vi "string array manage.vi"(6 "pattern IN":string=".+?\\(.+?\\)", 7 "actions":T1=enum."match pattern", 9 "Array 2 IN":string[](array[string])=["frequency (Hz)", "Cs/T (J/K^2)", "Ts (K)", "Tr (K)", "Cs (J/K)", "Cr (J/K)", "Ks (W/K)", "Kr (W/K)", "Rs-therm (Ohm)", "Rr-therm (Ohm)", "Cr/T (J/K^2)", "dlogR/dlogT -- S  (a.u.)", "tau (s)", "tan(phi) (a.u)", "Ts,ac (K)", "Tr,ac (K)", "Hs,ac,out (V)", "Offset,dc,out (V)", "Stherm,ac,out (V)", "Rtherm,ac,out (V)", "CV1 -- Re (V)", "CV1 -- Im (V)", "DV2 -- Re (V)", "DV2 -- Im (V)", "AV2 -- Re (V)", "AV2 -- Im (V)", "LakeShore 336 (12) A", "LakeShore 336 (12) B", "LakeShore 336 (12) C", "LakeShore 336 (12) D", "field (T)"], 10 "Array 1 IN":string[](array[string])=["Time", "frequency (Hz)", "Cs/T (J/K^2)", "Ts (K)", "Tr (K)", "Cs (J/K)", "Cr (J/K)", "Ks (W/K)", "Kr (W/K)", "Rs-therm (Ohm)", "Rr-therm (Ohm)", "Cr/T (J/K^2)", "dlogR/dlogT -- S  (a.u.)", "tau (s)", "tan(phi) (a.u)", "Ts,ac (K)", "Tr,ac (K)", "Hs,ac,out (V)", "Offset,dc,out (V)", "Stherm,ac,out (V)", "Rtherm,ac,out (V)", "CV1 -- Re (V)", "CV1 -- Im (V)", "DV2 -- Re (V)", "DV2 -- Im (V)", "AV2 -- Re (V)", "AV2 -- Im (V)", "LakeShore 336 (12) A", "LakeShore 336 (12) B", "LakeShore 336 (12) C", "LakeShore 336 (12) D", "pos", "field (T)"]) -> (1 "Array 2 OUT":string[](array[string]), 2 "Array 1 OUT":string[](array[string])=["frequency (Hz)", "Cs/T (J/K^2)", "Ts (K)", "Tr (K)", "Cs (J/K)", "Cr (J/K)", "Ks (W/K)", "Kr (W/K)", "Rs-therm (Ohm)", "Rr-therm (Ohm)", "Cr/T (J/K^2)", "dlogR/dlogT -- S  (a.u.)", "tau (s)", "tan(phi) (a.u)", "Ts,ac (K)", "Tr,ac (K)", "Hs,ac,out (V)", "Offset,dc,out (V)", "Stherm,ac,out (V)", "Rtherm,ac,out (V)", "CV1 -- Re (V)", "CV1 -- Im (V)", "DV2 -- Re (V)", "DV2 -- Im (V)", "AV2 -- Re (V)", "AV2 -- Im (V)", "LakeShore 336 (12) A", "LakeShore 336 (12) B", "LakeShore 336 (12) C", "LakeShore 336 (12) D", "field (T)"])   [LabVIEW 2021]
uses:
  string array manage control.ctl
  6d6d019a-d48c-a744-8711-00c2e699bb64.vi
  <vilib>/regexp/Match Regular Expression.xnode
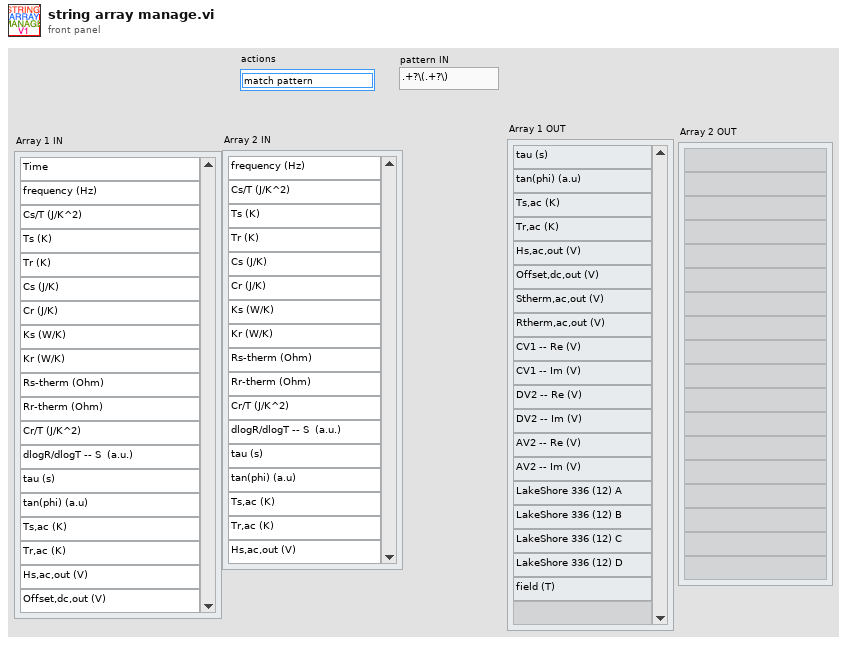
[diagram p1: front panel]
types:
  T1 = typedef "string array manage control.ctl" = enum16{"intersection", "match pattern"}
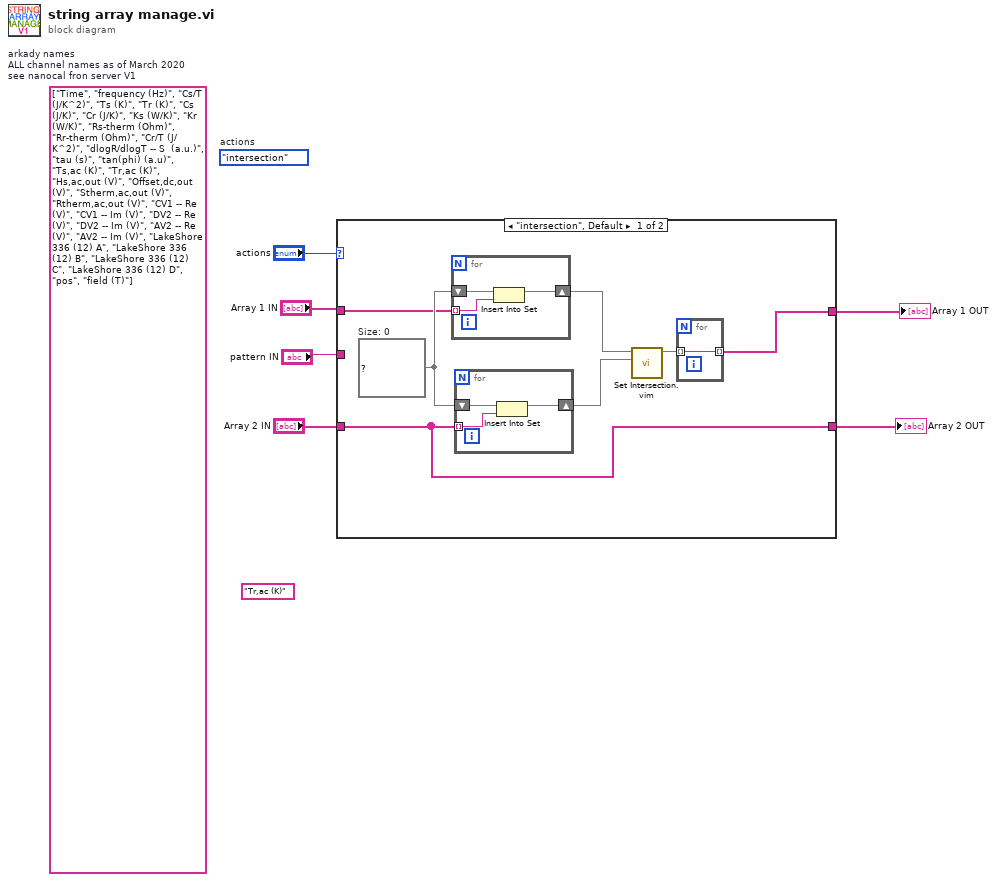
[diagram p0: block diagram]
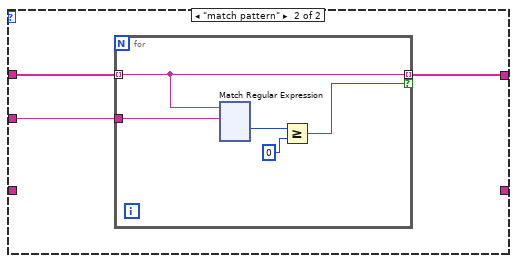
[diagram p2: hidden frame]
diagram:
  (unwired) "Tr,ac (K)"
  (unwired) string_array_manage_control."intersection"  # actions
  (unwired) string[] ["Time", "frequency (Hz)", "Cs/T (J/K^2)", "Ts (K)", "Tr (K)", "Cs (J/K)", "Cr (J/K)", "Ks (W/K)", "Kr (W/K)", "Rs-therm (Ohm)", "Rr-therm (Ohm)", "Cr/T (J/K^2)", "dlogR/dlogT -- S  (a.u.)", "tau (s)", "tan(phi) (a.u)", "Ts,ac (K)", "Tr,ac (K)", "Hs,ac,out (V)", "Offset,dc,out (V)", "Stherm,ac,out (V)", "Rtherm,ac,out (V)", "CV1 -- Re (V)", "CV1 -- Im (V)", "DV2 -- Re (V)", "DV2 -- Im (V)", "AV2 -- Re (V)", "AV2 -- Im (V)", "LakeShore 336 (12) A", "LakeShore 336 (12) B", "LakeShore 336 (12) C", "LakeShore 336 (12) D", "pos", "field (T)"]  # arkady names ALL channel names as of March 2020 see nanocal fron server V1
  n1 = case shown="\"intersection\", Default" "actions" {
    tunnel: "Array 2 IN" -> [w7 _]
    tunnel: "Array 1 IN" -> [w12 w23]
    tunnel: [w8 w21] -> w3
    tunnel: "pattern IN" -> [_ w22]
    tunnel: [w7 _] -> w1
    frame "intersection", Default {
      w13 = set{string} {}  # Size: 0
      n2 = for {
        tunnel: w12 -> [w17] mode=indexing
        shift-right: [w15] -> w11
        shift-left: w13 -> [w16]
        n3 = Insert Into Set(10:w17, 11:w16) -> (3:w15:set{string})  [unwired: 1 out]
      }
      n4 = for {
        tunnel: w7 -> [w18] mode=indexing
        shift-right: [w19] -> w10
        shift-left: w13 -> [w20]
        n5 = Insert Into Set(10:w18, 11:w20) -> (3:w19:set{string})  [unwired: 1 out]
      }
      n6 = call "Set Intersection.vim"("set 2"=w10, "set 1"=w11) -> ("intersection"=w9:set{string})  [unwired: 9 in]
      n7 = for {
        tunnel: w9 -> [w14] mode=indexing
        tunnel: [w14] -> w8 mode=indexing
      }
    }
    frame "match pattern" {
      n8 = for {
        tunnel: w23 -> [w25] mode=indexing
        tunnel: w22 -> [w28]
        tunnel: [w25] -> w21 mode=indexing if=w24
        n9 = xnode "Match Regular Expression"("input string"=w25, "regular expression"=w28) -> ("offset past match"=w27:i32)  [unwired: 4 in, 4 out]
        n10 = Greater Or Equal?(x=w27, y=0) -> (x >= y?=w24:bool)
      }
    }
  }
  "Array 1 OUT" <- w3
  "Array 2 OUT" <- w1
